vi "leftShifText.vi"(8 "error in (no error)":errorcluster, 9 "textIn":string, 10 "numberOfLoops":i32, 11 "TextDisplay Class in":refnum<class "TextDisplay Class.lvclass">) -> (0 "error out":errorcluster, 3 "TextDisplay Class out":refnum<class "TextDisplay Class.lvclass">)   [LabVIEW 2019, in "TextDisplay Class.lvclass"]
uses:
  TextDisplay Class.lvclass
  TextDisplay Class.lvclass/TextDisplay Class.ctl
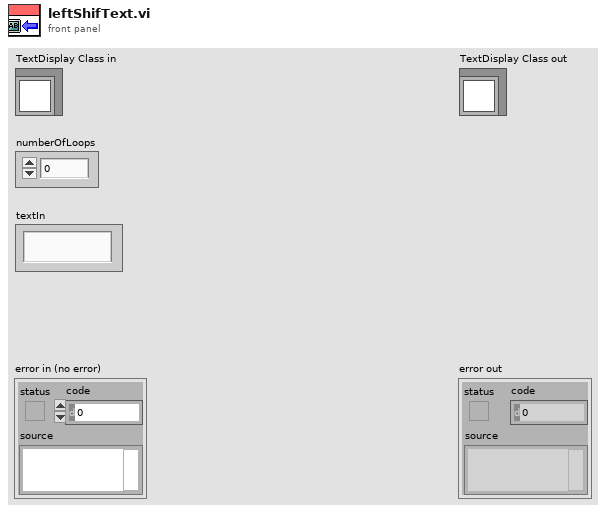
[diagram p1: front panel]
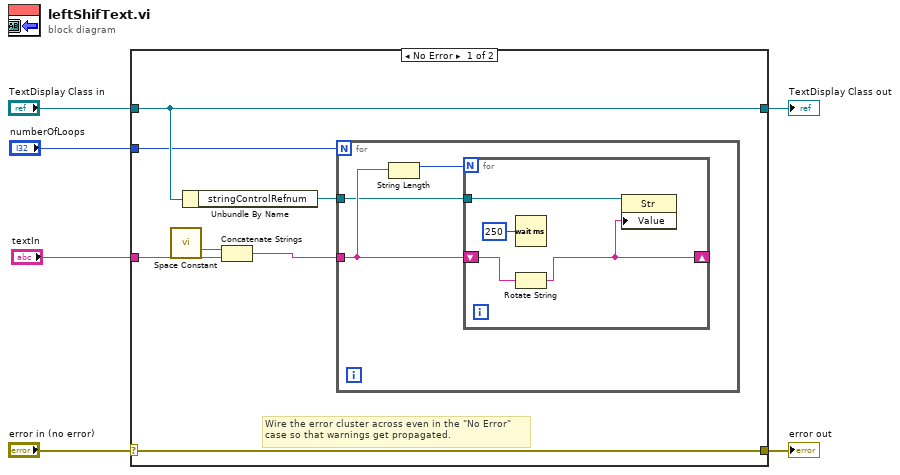
[diagram p0: block diagram]
diagram:
  n1 = case shown="No Error" "error in (no error)" {
    selector: "error in (no error)" -> [w13 w22]
    tunnel: [w13 w22] -> w5
    tunnel: [w12 w21] -> w3
    tunnel: "TextDisplay Class in" -> [w12 w21]
    tunnel: "textIn" -> [w11 _]
    tunnel: "numberOfLoops" -> [w9 _]
    frame No Error {
      # "Wire the error cluster across even in the \"No Error\"\ncase so that warnings get propagated."
      n2 = call <vilib>:"Space Constant.vi"() -> ("String"=w7:string)
      n3 = Unbundle By Name(w12) -> ("stringControlRefnum"=w10:refnum<vi>)
      n4 = Concatenate Strings(w7, w11) -> (w8:string)
      n5 = for {
        N: w9 -> [_]
        tunnel: w8 -> [w15]
        tunnel: w10 -> [w14]
        n6 = String Length(string=w15) -> (length=w16:i32)
        n7 = for {
          N: w16 -> [_]
          shift-right: [w17] -> _
          shift-left: w15 -> [w20]
          tunnel: w14 -> [w18]
          n8 = Wait (ms)(milliseconds to wait=u32 250) -> ()  [unwired: 1 out]
          n9 = Rotate String(1:w20) -> (0:w17:string)
          n10 = property class="Str"(reference=w18, "Value"=w17) -> ()  [unwired: 1 in, 2 out]
        }
      }
    }
    frame Error {
    }
  }
  "error out" <- w5
  "TextDisplay Class out" <- w3
